vi "fits2ds9.vi"(8 "DS9path":path, 11 "FitsFile":path) -> ()   [LabVIEW 2011]
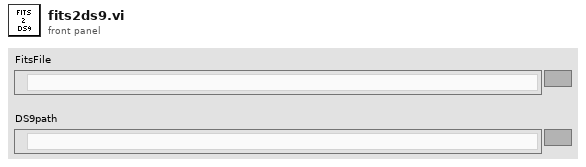
[diagram p1: front panel]
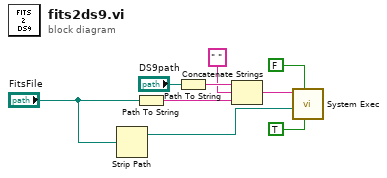
[diagram p0: block diagram]
diagram:
  n1 = Strip Path(path="FitsFile") -> (stripped path=w1:path)  [unwired: 1 out]
  n2 = Path To String(path="FitsFile") -> (string=w7:string)
  n3 = Path To String(path="DS9path") -> (string=w8:string)
  n4 = Concatenate Strings(w8, " " ("string"), w7) -> (w5:string)
  n5 = call <vilib>:"System Exec.vi"("run minimized? (F)"=TRUE, "wait until completion? (T)"=FALSE, "working directory"=w1, "command line"=w5) -> ()  [unwired: 4 in, 4 out]
